vi "Read Scratchpad.vi"(6 "1-Wire DIO Pin":refnum<k21>="ConnectorA/DIO15", 7 "error in (no error)":errorcluster) -> (0 "error out":errorcluster, 2 "Scratchpad Data":u8[](array[numeric]) format="%.0x")   [LabVIEW 2014, in "Maxim 1-Wire.lvlib"]
doc: "READ SCRATCHPAD [BEh]\nThis command allows the master to read the contents of the scratchpad. The data transfer starts with the least significant bit of byte 0 and continues through the scratchpad until the 9th byte (byte 8 ? CRC) is read. The master may issue a reset to terminate reading at any time if only part of the scratchpad data is needed."
uses:
  Maxim 1-Wire.lvlib
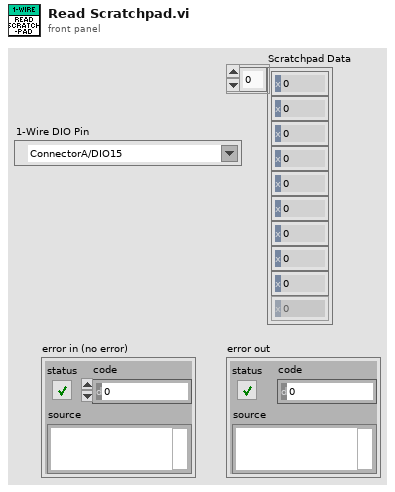
[diagram p1: front panel]
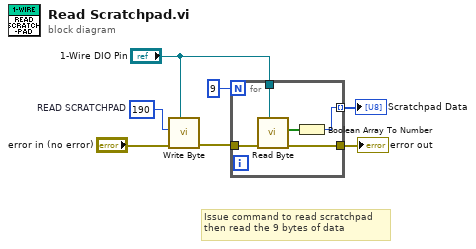
[diagram p0: block diagram]
diagram:
  w7 = u8 190  # READ SCRATCHPAD
  # "Issue command to read scratchpad\nthen read the 9 bytes of data"
  n1 = call "Write Byte.vi"("1-Wire DIO Pin"="1-Wire DIO Pin", "error in"="error in (no error)", "Tx data"=w7) -> ("error out"=w4:errorcluster)  [unwired: 8 in]
  n2 = for {
    N: 9 -> [_]
    tunnel: w4 -> [w12]
    tunnel: [w11] -> w6
    tunnel: [w9] -> w2 mode=indexing
    tunnel: "1-Wire DIO Pin" -> [w8]
    n3 = call "Read Byte.vi"("1-Wire DIO Pin"=w8, "error in"=w12) -> ("error out"=w11:errorcluster, "Bit Array"=w10:bool[])  [unwired: 8 in]
    n4 = Boolean Array To Number(Boolean array=w10) -> (number=w9:u8)
  }
  "Scratchpad Data" <- w2
  "error out" <- w6
